vi "Change Bookmark View.vi"(8 "Error In":errorcluster, 10 "Data":variant, 11 "State In":T1) -> (0 "Error Out":errorcluster, 3 "State Out":T1)   [LabVIEW 2017, in "Graveyard.lvlib"]
uses:
  Graveyard.lvlib
  State.ctl
  Bookmarks Views.ctl
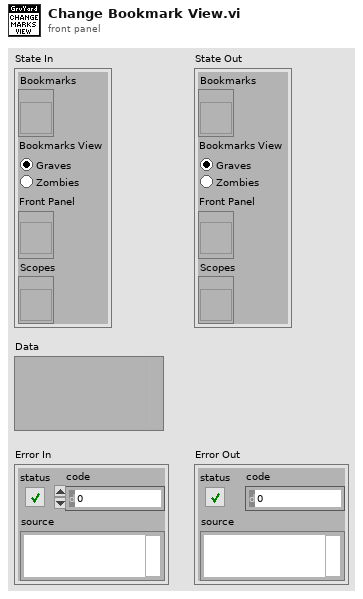
[diagram p1: front panel]
types:
  T1 = typedef "Graveyard.lvlib/State.ctl" = cluster{"Bookmarks":refnum<vi>, "Bookmarks View":T2, "Front Panel":refnum<vi>, "Scopes":refnum<vi>}
  T2 = typedef "Graveyard.lvlib/Bookmarks Views.ctl" = enum32{"Graves", "Zombies"}
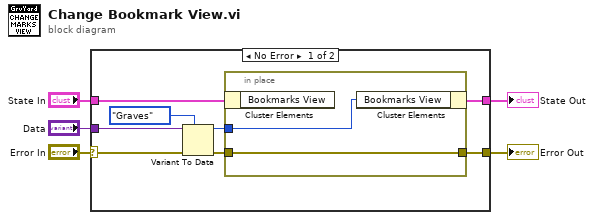
[diagram p0: block diagram]
diagram:
  n1 = case shown="No Error" "Error In" {
    selector: "Error In" -> [w8 w16]
    tunnel: [w11 w17] -> w5
    tunnel: "State In" -> [w10 w17]
    tunnel: "Data" -> [w9 _]
    tunnel: [w6 w16] -> w2
    frame No Error {
      n2 = Variant To Data(error in=w8, type=Bookmarks_Views."Graves" ("Bookmarks Type"), Variant=w9) -> (data=w12:T2, error out=w7:errorcluster)
      n3 = in-place {
        in-place-border: w12 -> [w15]
        in-place-border: w7 -> [w14]
        in-place-border: [w14] -> w6
        n4 = in-place-cluster #1(w10) -> ()  [unwired: 1 out]
        n5 = in-place-cluster #1("Bookmarks View"=w15) -> (w11:T1)
      }
    }
    frame Error {
    }
  }
  "State Out" <- w5
  "Error Out" <- w2
